vi "Configure.vi"(8 "error in (no error)":errorcluster, 11 "RSA in":refnum<class "RSA.lvclass">) -> (0 "error out":errorcluster, 2 "cancelled?":bool, 3 "RSA out":refnum<class "RSA.lvclass">)   [LabVIEW 2012, in "RSA.lvclass"]
doc: "The configure method configures the details for the RabbitMQ connection. \n\nIn the derived class, make a call to the parent for setting these parameters."
uses:
  RSA.lvclass
  <vilib>/Utility/miscctls.llb/LVPointTypeDef.ctl
  RSA.lvclass/RSA.ctl
  <vilib>/Distrio/Murmex/Murmex/Murmex.lvclass
panel:
  in  "button::ok":bool
  in  "button::configure murmex":bool
  in  "button::cancel":bool
  in  "Tab Control":enum32{"RSA", "Debug"}(tab)
  in  "initialised array":dbl[](array[numeric])
  # "RabbitMQ parameters"
  # "Window position"
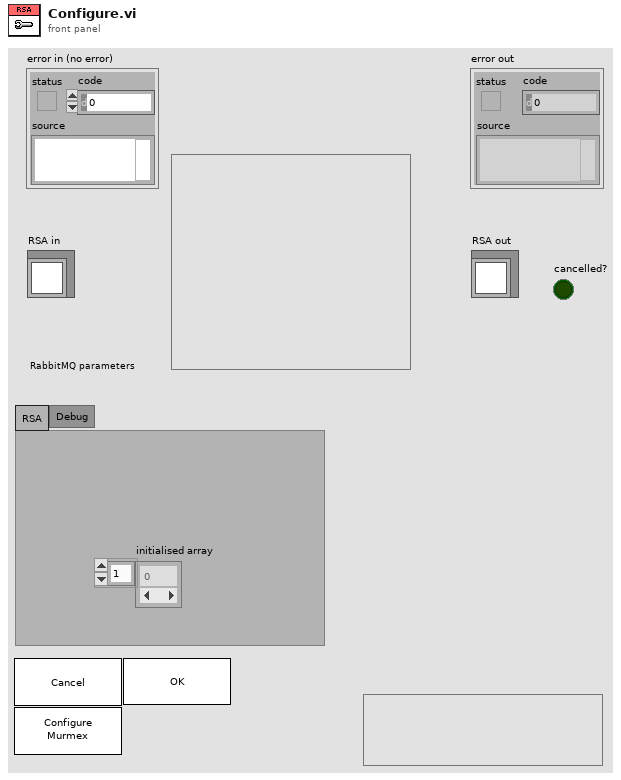
[diagram p1: front panel]
types:
  T1 = typedef "LVPointTypeDef.ctl" = cluster{"Horizontal":i16, "Vertical":i16}
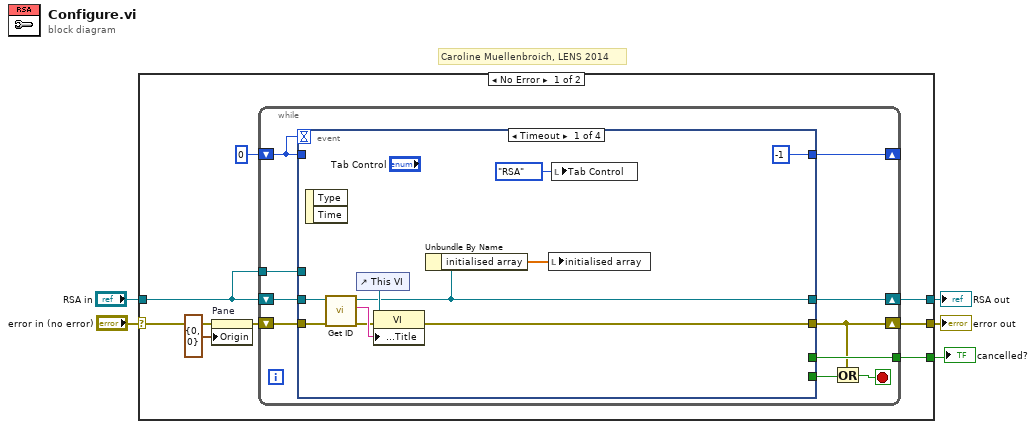
[diagram p0: block diagram]
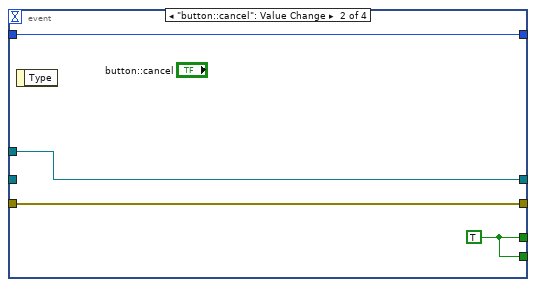
[diagram p2: hidden frame]
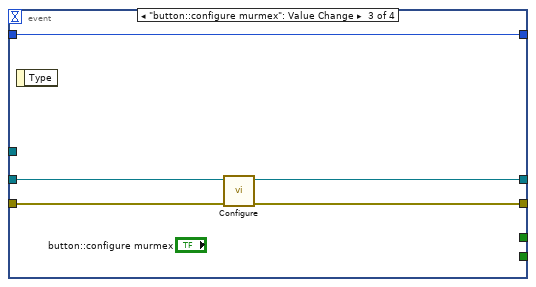
[diagram p3: hidden frame]
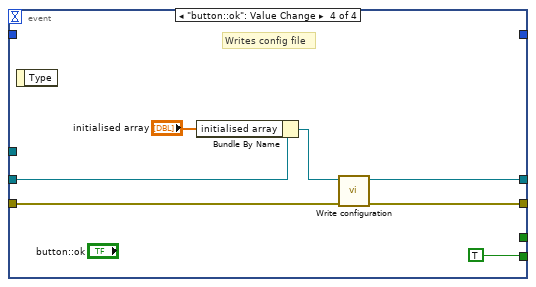
[diagram p4: hidden frame]
diagram:
  # "Caroline Muellenbroich, LENS 2014"
  n1 = case shown="No Error" "error in (no error)" {
    selector: "error in (no error)" -> [w13 w51]
    tunnel: "RSA in" -> [w10 w50]
    tunnel: [w8 w51] -> w3
    tunnel: [w7 w50] -> w2
    tunnel: [w6 _] -> w1
    frame No Error {
      n2 = property on="Pane" class="Pane"(error in=w13, "Origin"=T1 {"Horizontal"=0, "Vertical"=0}) -> (error out=w11:errorcluster)  [unwired: 1 in, 1 out]
      n3 = while {
        shift-right: [w20] -> w7
        shift-left: w10 -> [w21]
        shift-right: [w16] -> w8
        shift-left: w11 -> [w22]
        tunnel: w10 -> [w18]
        shift-right: [w19] -> _
        shift-left: 0 -> [w23]
        tunnel: [w17] -> w6
        stop <- w14 stop-if-true
        n4 = event shown="[0] Timeout" {
          selector: _ -> [_ _ _ _]
          dyn-events: _ -> [_ _ _ _]
          timeout: w23 -> [_ _ _ _]
          tunnel: w23 -> [_ w37 w42 _]
          tunnel: w22 -> [w30 w36 w41 w48]
          tunnel: w21 -> [w29 _ w39 w45]
          tunnel: [w25 w35 w38 w46] -> w20
          tunnel: [w28 w36 w40 w47] -> w16
          tunnel: [-1 w37 w42 _] -> w19
          tunnel: w18 -> [_ w35 _ _]
          tunnel: [_ w34 _ _] -> w17
          tunnel: [_ w34 _ TRUE ("force loading?")] -> w15
          event Timeout {
            n5 = event-data() -> ()  [unwired: 1 in, 2 out]
            n6 = call <vilib>:"Get ID.vi"("error in (no error)"=w30, "Murmex in"=w29) -> ("error out"=w32:errorcluster, "component id"=w33:string, "Murmex out"=w25:refnum<class "RSA.lvclass">)  [unwired: 7 in]
            n7 = control-ref of="This VI"() -> (w31:refnum<vi>)
            n8 = property class="VI"(reference=w31, error in=w32, "Front Panel.Title"=w33) -> (error out=w28:errorcluster)  [unwired: 1 out]
            n9 = Unbundle By Name(w25) -> ("initialised array"=w24:dbl[])
            n10 = local write "initialised array"(w24) -> ()
            n11 = local write "Tab Control"(enum32{"RSA", "Debug"}."RSA" ("Tab Control")) -> ()
          }
          event "button::cancel": Value Change {
            w34 = TRUE ("force loading?")
            n12 = event-data() -> ()  [unwired: 1 in, 1 out]
          }
          event "button::configure murmex": Value Change {
            n13 = event-data() -> ()  [unwired: 1 in, 1 out]
            n14 = call-parent "Configure.vi"("error in (no error)"=w41, "Murmex in"=w39) -> ("error out"=w40:errorcluster, "Murmex out"=w38:refnum<class "RSA.lvclass">)  [unwired: 7 in, 1 out]
          }
          event "button::ok": Value Change {
            # "Writes config file"
            n15 = event-data() -> ()  [unwired: 1 in, 1 out]
            n16 = Bundle By Name(cluster=w45, "initialised array"="initialised array") -> (w44:refnum<class "RSA.lvclass">)
            n17 = call-dynamic "Write configuration.vi"("error in (no error)"=w48, "RSA in"=w44) -> ("error out"=w47:errorcluster, "RSA out"=w46:refnum<class "RSA.lvclass">)  [unwired: 8 in]
          }
        }
        n18 = Or(x=w16, y=w15) -> (x .or. y?=w14:bool)
      }
    }
    frame Error {
    }
  }
  "error out" <- w3
  "RSA out" <- w2
  "cancelled?" <- w1
